vi "Set Stage Speed.vi"(8 "error in (no error)":errorcluster, 9 "Y Axis":dbl, 10 "X Axis":dbl, 11 "2-Axis Stage in":refnum<class "2-Axis Stage Actions.lvclass">) -> (0 "error out":errorcluster, 3 "2-Axis Stage out":refnum<class "2-Axis Stage Actions.lvclass">)   [LabVIEW 2022 SP3, in "2-Axis Stage Actions.lvclass"]
uses:
  2-Axis Stage Actions.lvclass
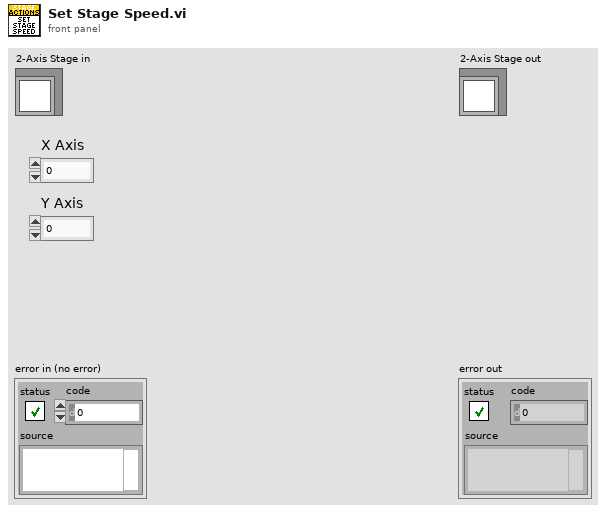
[diagram p1: front panel]
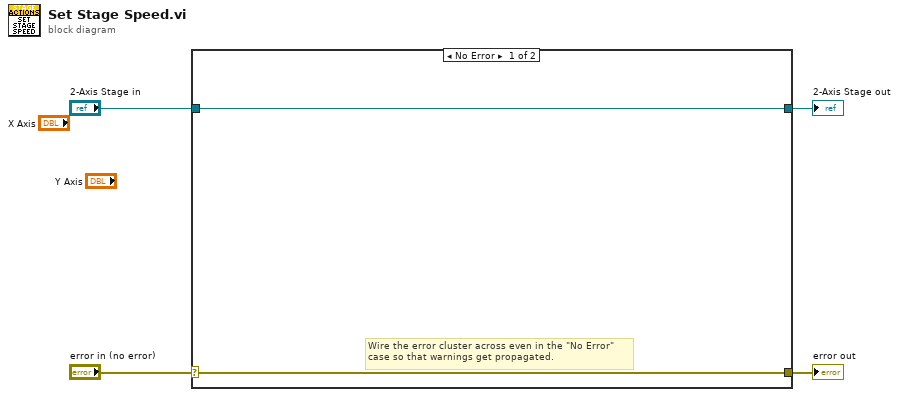
[diagram p0: block diagram]
diagram:
  n1 = case shown="No Error" "error in (no error)" {
    selector: "error in (no error)" -> [w5 w8]
    tunnel: [w5 w8] -> w3
    tunnel: [w6 w7] -> w1
    tunnel: "2-Axis Stage in" -> [w6 w7]
    frame No Error {
      # "Wire the error cluster across even in the \"No Error\"\ncase so that warnings get propagated."
    }
    frame Error {
    }
  }
  "error out" <- w3
  "2-Axis Stage out" <- w1
